vi "String Contents Fit.vi"(8 "error in (no error)":errorcluster, 11 "String":refnum<vi>) -> (0 "error out":errorcluster, 3 "dup String":refnum<vi>)   [LabVIEW 2016]
panel:
  out "Temporary":string
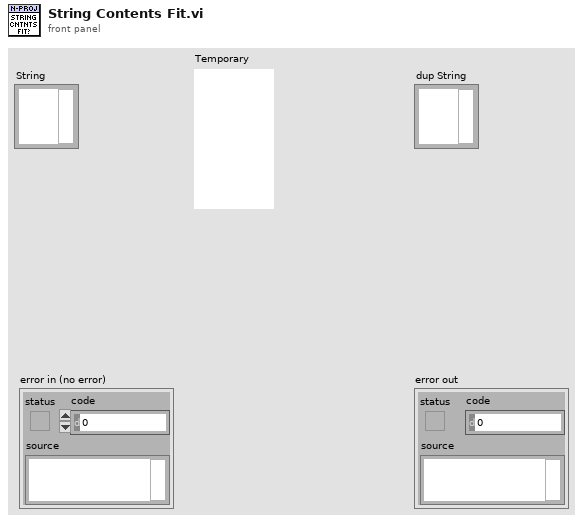
[diagram p1: front panel]
types:
  T1 = typedef "LVBoundsTypeDef.ctl" = cluster{"Width":u32, "Height":u32}
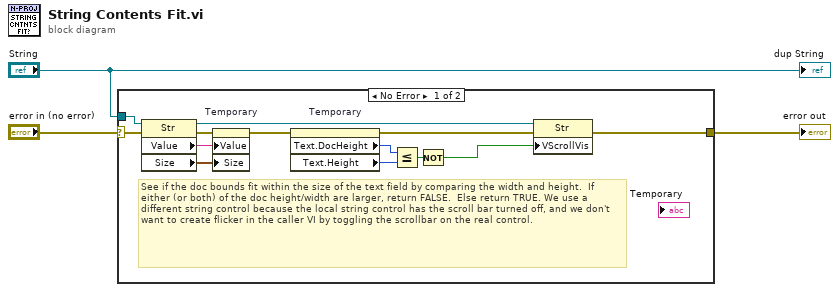
[diagram p0: block diagram]
diagram:
  n1 = case shown="No Error" "error in (no error)" {
    selector: "error in (no error)" -> [w9 w17]
    tunnel: "String" -> [w14 _]
    tunnel: [w6 w17] -> w2
    frame No Error {
      # "See if the doc bounds fit within the size of the text field by comparing the width and height.  If either (or both) of the doc height/width are larger, return FALSE.  Else return TRUE. We use a different string control because the local string control has the scroll bar turned off, and we don't want to create flicker in the caller VI by toggling the scrollbar on the real control."
      n2 = property class="Str"(reference=w14, error in=w9) -> (reference out=w4:refnum<vi>, error out=w11:errorcluster, "Value"=w13:string, "Size"=w12:T1)
      n3 = property on="Temporary" class="Str"(error in=w11, "Value"=w13, "Size"=w12) -> (error out=w10:errorcluster)  [unwired: 1 in, 1 out]
      n4 = property on="Temporary" class="Str"(error in=w10) -> (error out=w7:errorcluster, "Text.DocHeight"=w16:u32, "Text.Height"=w15:u32)  [unwired: 1 in, 1 out]
      n5 = Less Or Equal?(x=w16, y=w15) -> (x <= y?=w8:bool)
      n6 = Not(x=w8) -> (.not. x?=w5:bool)
      n7 = property on="Property Node" class="Str"(reference=w4, error in=w7, "VScrollVis"=w5) -> (error out=w6:errorcluster)  [unwired: 1 out]
    }
    frame Error {
    }
  }
  "error out" <- w2
  "dup String" <- "String"
